vi "Add Command.vi"(8 "error in (no error)":errorcluster, 10 "Settings":T1 {"Linkages"."Channel Ref" format="%.0x"}, 11 "Message Refnum In":T4 format="%.0x") -> (0 "error out":errorcluster, 2 "Command Refnum":T4 format="%.0x", 3 "Message Refnum Out":T4 format="%.0x")   [LabVIEW 2018, in "Instrument Addon Scripting API.lvlib"]
uses:
  Instrument Addon Scripting API.lvlib
  <vilib>/NI Veristand/Custom Device API/Custom Device Item Ref.ctl
  TypeDefs/Command Settings.ctl
  TypeDefs/Padding.ctl
  TypeDefs/Linked Channel.ctl
  Addon/Addon Shared/SubVIs/Constants.vi
  <vilib>/NI Veristand/Custom Device API/Set Item Property (String).vi
  <vilib>/NI Veristand/Custom Device API/Set Item Property (String Array).vi
  <vilib>/NI Veristand/Custom Device API/Set Item Property (Boolean).vi
  <vilib>/NI Veristand/Custom Device API/Set Item Property (U32).vi
  Addon/Addon Shared/Instrument Addon Shared.lvlib
  <vilib>/NI VeriStand/Custom Device API/Custom Device API.lvlib
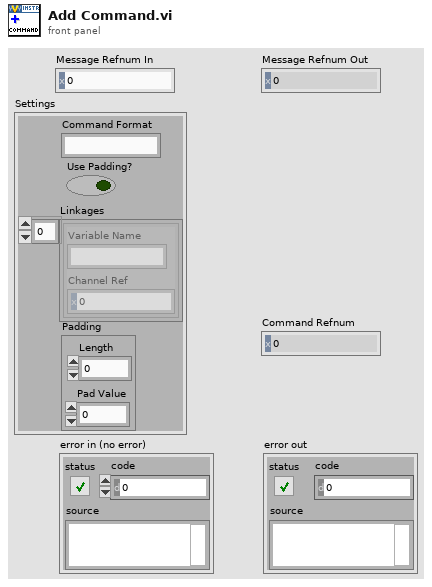
[diagram p1: front panel]
types:
  T1 = typedef "Instrument Addon Scripting API.lvlib/Command Settings.ctl" = cluster{"Command Format":string, "Use Padding?":bool, "Padding":T2, "Linkages":T3}
  T2 = typedef "Instrument Addon Scripting API.lvlib/Padding.ctl" = cluster{"Length":u32, "Pad Value":u8}
  T3 = typedef "Instrument Addon Scripting API.lvlib/Linked Channel.ctl" = cluster{"Channel Ref":T4, "Variable Name":string}[]
  T4 = typedef "Custom Device API.lvlib/Custom Device Item Ref.ctl" = u64
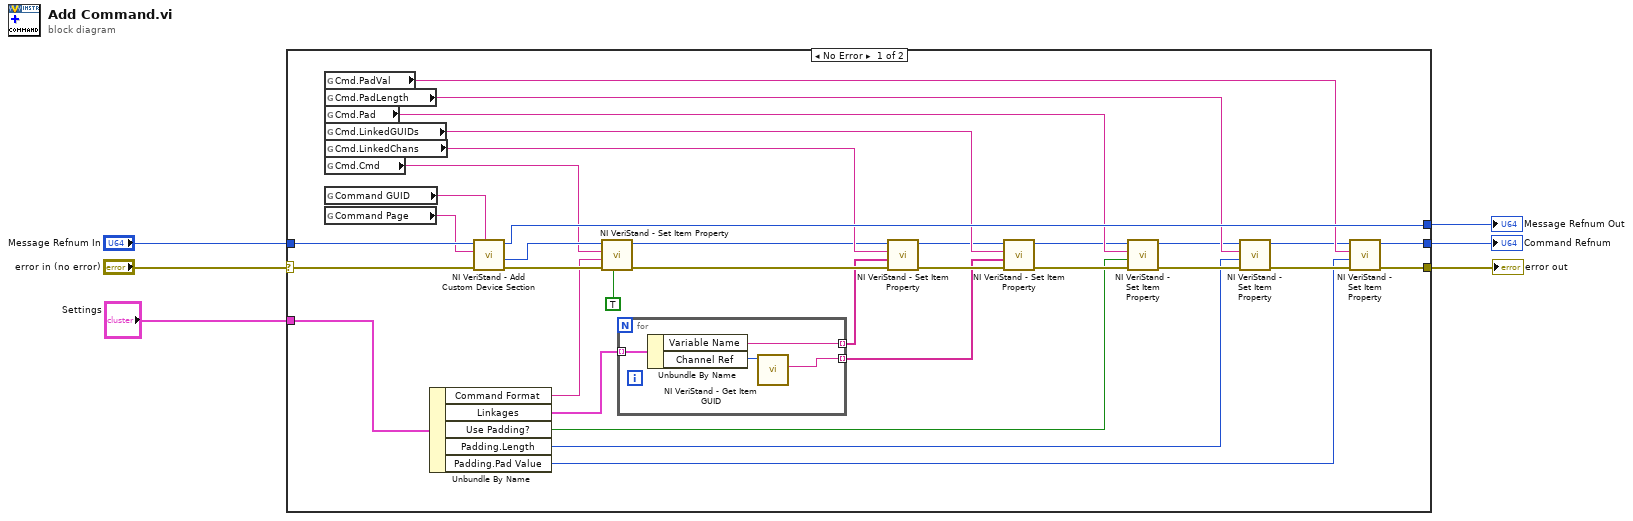
[diagram p0: block diagram]
diagram:
  n1 = case shown="No Error" "error in (no error)" {
    selector: "error in (no error)" -> [w36 w46]
    tunnel: "Message Refnum In" -> [w40 w45]
    tunnel: [w39 w45] -> w5
    tunnel: [w32 w46] -> w4
    tunnel: [w33 _] -> w2
    tunnel: "Settings" -> [w31 _]
    frame No Error {
      n2 = global read "Constants.vi" "Cmd.PadVal"() -> (w30:string)
      n3 = global read "Constants.vi" "Cmd.PadLength"() -> (w29:string)
      n4 = global read "Constants.vi" "Cmd.Pad"() -> (w28:string)
      n5 = global read "Constants.vi" "Cmd.LinkedGUIDs"() -> (w27:string)
      n6 = global read "Constants.vi" "Cmd.LinkedChans"() -> (w26:string)
      n7 = global read "Constants.vi" "Cmd.Cmd"() -> (w25:string)
      n8 = global read "Constants.vi" "Command GUID"() -> (w37:string)
      n9 = global read "Constants.vi" "Command Page"() -> (w38:string)
      n10 = Unbundle By Name(w31) -> ("Command Format"=w24:string, "Linkages"=w22:T3, "Use Padding?"=w9:bool, "Padding.Length"=w8:u32, "Padding.Pad Value"=w7:u8)
      n11 = call <vilib>:"NI VeriStand - Add Custom Device Section.vi"("GUID (Default Section)"=w37, "error in (no error)"=w36, "Section Name"=w38, "Parent Ref in"=w40) -> ("error out"=w35:errorcluster, "Section Ptr"=w34:T4, "Parent Ref out"=w39:T4)  [unwired: 4 in, 1 out]
      n12 = call-poly <vilib>:"NI VeriStand - Set Item Property.vi"("Binary String (T)"=TRUE, "error in (no error)"=w35, "Value"=w24, "Property Name"=w25, "Item Ref in"=w34) -> ("error out"=w20:errorcluster, "Item Ref out"=w21:T4)  [unwired: 4 in, 1 out]
      n13 = for {
        tunnel: w22 -> [w44] mode=indexing
        tunnel: [w43] -> w10 mode=indexing
        tunnel: [w41] -> w11 mode=indexing
        n14 = Unbundle By Name(w44) -> ("Variable Name"=w43:string, "Channel Ref"=w42:T4)
        n15 = call <vilib>:"NI VeriStand - Get Item GUID.vi"("Item Ref in"=w42) -> ("GUID"=w41:string)  [unwired: 8 in, 2 out]
      }
      n16 = call-poly <vilib>:"NI VeriStand - Set Item Property.vi"("error in (no error)"=w20, "Value"=w10, "Property Name"=w26, "Item Ref in"=w21) -> ("error out"=w19:errorcluster, "Item Ref out"=w12:T4)  [unwired: 5 in, 1 out]
      n17 = call-poly <vilib>:"NI VeriStand - Set Item Property.vi"("error in (no error)"=w19, "Value"=w11, "Property Name"=w27, "Item Ref in"=w12) -> ("error out"=w18:errorcluster, "Item Ref out"=w13:T4)  [unwired: 5 in, 1 out]
      n18 = call-poly <vilib>:"NI VeriStand - Set Item Property.vi"("error in (no error)"=w18, "Value"=w9, "Property Name"=w28, "Item Ref in"=w13) -> ("error out"=w17:errorcluster, "Item Ref out"=w14:T4)  [unwired: 5 in, 1 out]
      n19 = call-poly <vilib>:"NI VeriStand - Set Item Property.vi"("error in (no error)"=w17, "Value"=w8, "Property Name"=w29, "Item Ref in"=w14) -> ("error out"=w16:errorcluster, "Item Ref out"=w15:T4)  [unwired: 5 in, 1 out]
      n20 = call-poly <vilib>:"NI VeriStand - Set Item Property.vi"("error in (no error)"=w16, "Value"=w7, "Property Name"=w30, "Item Ref in"=w15) -> ("error out"=w32:errorcluster, "Item Ref out"=w33:T4)  [unwired: 5 in, 1 out]
    }
    frame Error {
    }
  }
  "Message Refnum Out" <- w5
  "error out" <- w4
  "Command Refnum" <- w2
